vi "Test Reading Output to Serial 0.vi"   [LabVIEW 2014, in "Arduino SoftwareSerial Wrapper.lvlib"]
uses:
  Arduino SoftwareSerial Wrapper.lvlib
  <vilib>/Aledyne-TSXperts/Arduino Compatible Compiler for LabVIEW/Code Generator/Arduino APIs/Serial/Serial Settings.ctl
  <vilib>/Aledyne-TSXperts/Arduino Compatible Compiler for LabVIEW/Arduino Compatible Compiler for LabVIEW.lvlib
types:
  T1 = typedef "Arduino Compatible Compiler for LabVIEW.lvlib/Serial Settings.ctl" = u16
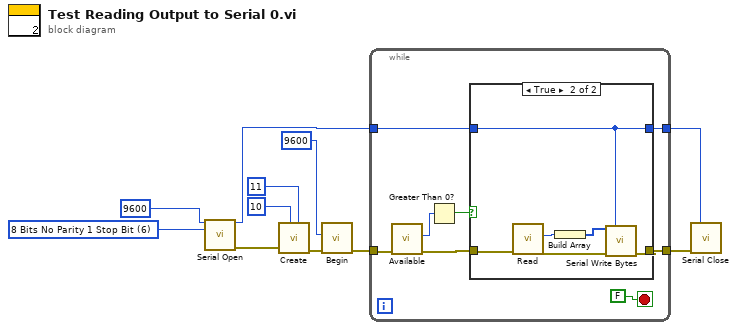
[diagram p0: block diagram]
diagram:
  w10 = T1 6 items=["5 Bits No Parity 1 Stop Bit"=0, "6 Bits No Parity 1 Stop Bit"=2, "7 Bits No Parity 1 Stop Bit"=4, "8 Bits No Parity 1 Stop Bit"=6, "5 Bits No Parity 2 Stop Bits"=8, "6 Bits No Parity 2 Stop Bits"=10, "7 Bits No Parity 2 Stop Bits"=12, "8 Bits No Parity 2 Stop Bits"=14, "5 Bits Even Parity 1 Stop Bits"=32, "6 Bits Even Parity 1 Stop Bits"=34, "7 Bits Even Parity 1 Stop Bits"=36, "8 Bits Even Parity 1 Stop Bits"=38, "5 Bits Even Parity 2 Stop Bits"=40, "6 Bits Even Parity 2 Stop Bits"=42, "7 Bits Even Parity 2 Stop Bits"=44, "8 Bits Even Parity 2 Stop Bits"=46, "5 Bits Odd Parity 1 Stop Bits"=48, "6 Bits Odd Parity 1 Stop Bits"=50, "7 Bits Odd Parity 1 Stop Bits"=52, "8 Bits Odd Parity 1 Stop Bits"=54, "5 Bits Odd Parity 2 Stop Bits"=56, "6 Bits Odd Parity 2 Stop Bits"=58, "7 Bits Odd Parity 2 Stop Bits"=60, "8 Bits Odd Parity 2 Stop Bits"=62] ("Serial Settings")
  n1 = call <vilib>:"Serial Open.vi"("Speed"=u32 9600, "Serial Settings"=w10) -> ("Instance"=w8:u8, "error out"=w9:errorcluster)  [unwired: 12 in]
  n2 = call "Create.vi"("arduino RX pin"=u8 11 ("TX pin"), "arduino TX pin"=u8 10 ("RX pin"), "Error In"=w9) -> ("Error Out"=w7:errorcluster)  [unwired: 8 in]
  n3 = call "Begin.vi"("Error In"=w7, "Baudrate"=u16 9600) -> ("Error Out"=w6:errorcluster)  [unwired: 8 in]
  n4 = while {
    tunnel: w6 -> [w12]
    tunnel: w8 -> [w13]
    tunnel: [w14] -> w4
    tunnel: [w18] -> w3
    stop <- FALSE stop-if-true
    n5 = call "Available.vi"("Error In"=w12) -> ("Error Out"=w17:errorcluster, "Bytes to read"=w16:u16)  [unwired: 9 in]
    n6 = Greater Than 0?(x=w16) -> (x > 0?=w15:bool)
    n7 = case shown="True" w15 {
      tunnel: w17 -> [w21 w27]
      tunnel: w13 -> [w20 w26]
      tunnel: [w21 w23] -> w14
      tunnel: [w20 w26] -> w18
      frame False {
      }
      frame True {
        n8 = call "Read.vi"("Error In"=w27) -> ("Error Out"=w22:errorcluster, "Output char"=w25:u8)  [unwired: 9 in]
        n9 = Build Array(w25) -> (w24:u8[])
        n10 = call <vilib>:"Serial Write Bytes.vi"("Data"=w24, "Instance"=w26, "error in (no error)"=w22) -> ("error out"=w23:errorcluster)  [unwired: 12 in]
      }
    }
  }
  n11 = call <vilib>:"Serial Close.vi"("Instance"=w3, "error in (no error)"=w4) -> ()  [unwired: 13 in, 1 out]
